vi "SEND_ABC.vi"(1 "SEND_ARR":string) -> (0 "SEND_CHR":string)   [LabVIEW 2014]
panel:
  out "SEND_ARR":u8[](array[numeric])
  out "数组长度":i32
  out "Numeric 2":u8
  out "Numeric":u8
  out "Array":u16[](array[numeric])
  out "String":string
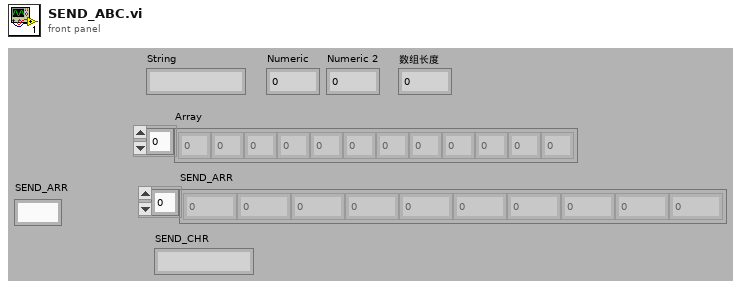
[diagram p1: front panel]
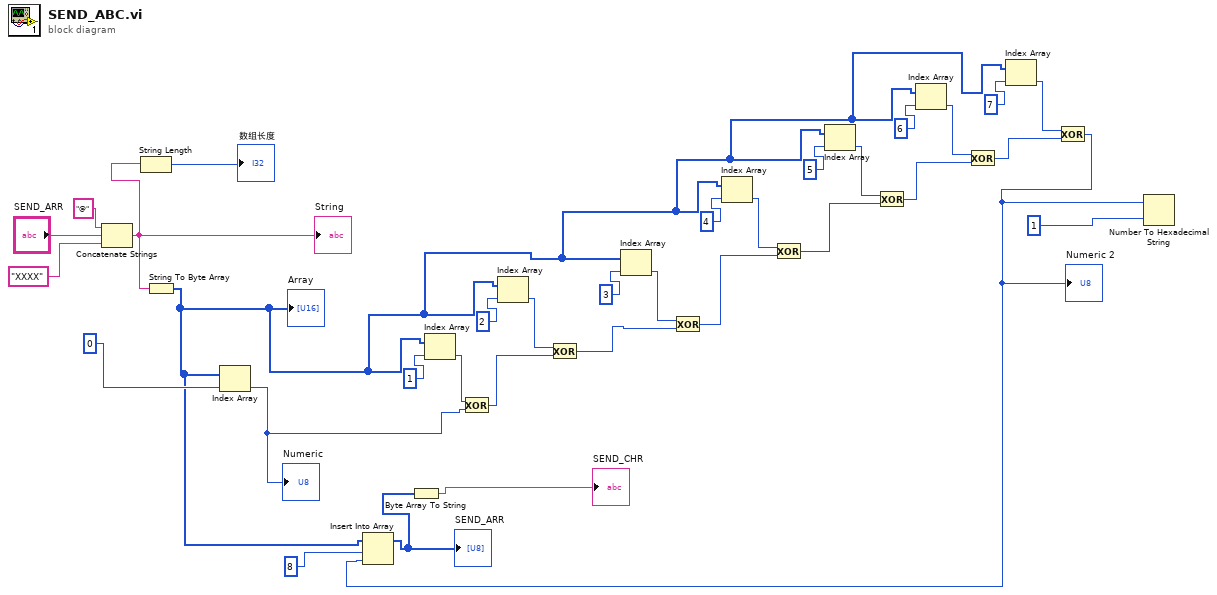
[diagram p0: block diagram]
diagram:
  n1 = Concatenate Strings("@", "SEND_ARR", "XXXX") -> (w3:string)
  "String" <- w3
  n2 = String Length(string=w3) -> (length=→"数组长度":i32)
  n3 = String To Byte Array(string=w3) -> (unsigned byte array=w6:u8[])
  "Array" <- w6
  n4 = Index Array(array=w6, index=0) -> (element=w25:u8)
  "Numeric" <- w25
  n5 = Index Array(array=w6, index=1) -> (element=w26:u8)
  n6 = Exclusive Or(1:w25, 2:w26) -> (0:w23:u8)
  n7 = Index Array(array=w6, index=2) -> (element=w22:u8)
  n8 = Exclusive Or(1:w23, 2:w22) -> (0:w19:u8)
  n9 = Index Array(array=w6, index=3) -> (element=w20:u8)
  n10 = Exclusive Or(1:w19, 2:w20) -> (0:w16:u8)
  n11 = Index Array(array=w6, index=4) -> (element=w17:u8)
  n12 = Exclusive Or(1:w16, 2:w17) -> (0:w13:u8)
  n13 = Index Array(array=w6, index=5) -> (element=w14:u8)
  n14 = Exclusive Or(1:w13, 2:w14) -> (0:w10:u8)
  n15 = Index Array(array=w6, index=6) -> (element=w11:u8)
  n16 = Exclusive Or(1:w10, 2:w11) -> (0:w7:u8)
  n17 = Index Array(array=w6, index=7) -> (element=w8:u8)
  n18 = Exclusive Or(1:w7, 2:w8) -> (0:w4:u8)
  "Numeric 2" <- w4
  n19 = Insert Into Array(array=w6, index=8, new element=w4) -> (w2:u8[])
  "SEND_ARR" <- w2
  n20 = Byte Array To String(unsigned byte array=w2) -> (string=→"SEND_CHR":string)
  n21 = Number To Hexadecimal String(1:1, 2:w4) -> ()  [unwired: 1 out]
